vi "Pockels Cal-Condition search.vi"(10 "Condition name":string, 11 "Pockels Cal table":string[](array[string])) -> (2 "Found?":bool, 3 "Index":i32)   [LabVIEW 2020]
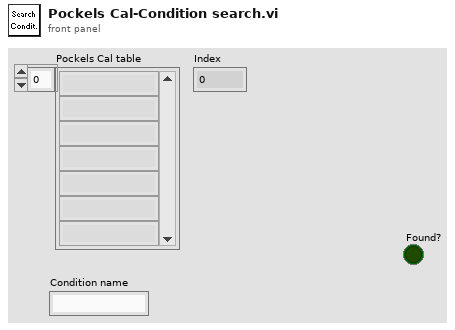
[diagram p1: front panel]
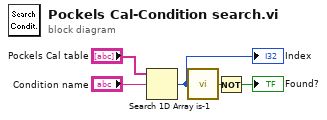
[diagram p0: block diagram]
diagram:
  n1 = Search 1D Array(1D array="Pockels Cal table", element="Condition name") -> (index of element=w4:i32)  [unwired: 1 in]
  "Index" <- w4
  n2 = call "is-1.vi"("Value"=w4) -> ("is -1?"=w3:bool)  [unwired: 4 in]
  n3 = Not(x=w3) -> (.not. x?=→"Found?":bool)
